vi "Draw Toolbar.vi"(8 "error in (no error)":errorcluster, 11 "Toolbar Control in":refnum<class "Toolbar Control.lvclass">) -> (0 "error out":errorcluster, 2 "Toolbar Image":picture, 3 "Toolbar Control out":refnum<class "Toolbar Control.lvclass">)   [LabVIEW 2011, in "Toolbar Control.lvclass"]
doc: "This VI will combine all the icons that are already drawn and return them on <B>Toolbar Image</B>.\n\n-------------\nDeveloped by Brian Hoover (hooovahh)"
uses:
  Toolbar Control.lvclass
  Toolbar Control.lvclass/Toolbar Control.ctl
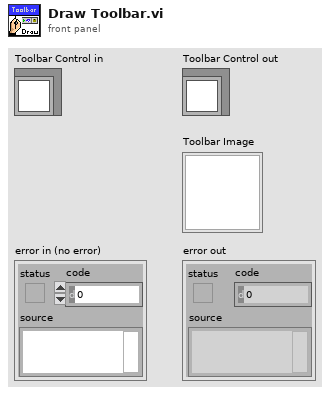
[diagram p1: front panel]
types:
  T1 = typedef "Toolbar Control.lvclass/Icon Data.ctl" = cluster{"Original Image Path":path, "Original Image Data":T2, "Scaled Icon":picture, "Button Name":string, "Button State":T3, "Icon Type":T4}
  T2 = typedef "imagedata.ctl" = cluster{"image type":i32, "image depth":i32, "image":u8[], "mask":u8[], "colors":u32[], "Rectangle":cluster{"left":i16, "top":i16, "right":i16, "bottom":i16}}
  T3 = typedef "Toolbar Control.lvclass/Button State.ctl" = enum8{"Enabled", "Disabled", "Disabled and Grayed Out"}
  T4 = typedef "Icon Type.ctl" = enum16{"Normal Icon", "Separator Icon", "More Options"}
  T5 = typedef "LVRectTypeDef.ctl" = cluster{"Left":i16, "Top":i16, "Right":i16, "Bottom":i16}
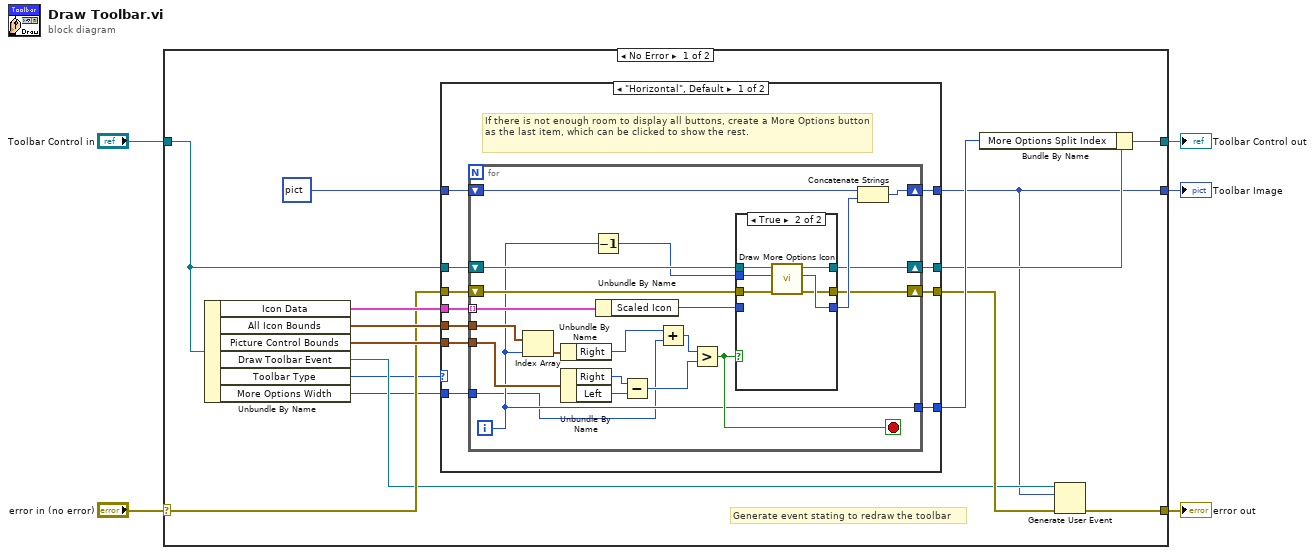
[diagram p0: block diagram]
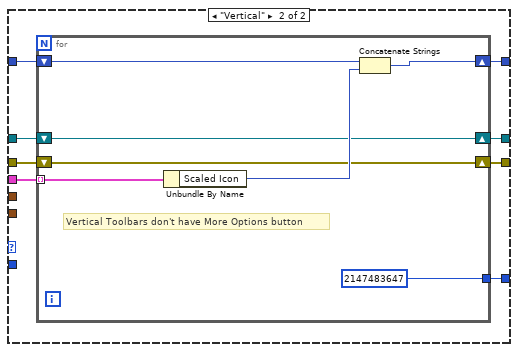
[diagram p3: hidden frame]
diagram:
  n1 = case shown="No Error" "error in (no error)" {
    selector: "error in (no error)" -> [w12 w78]
    tunnel: [w10 w78] -> w4
    tunnel: [w16 w77] -> w2
    tunnel: "Toolbar Control in" -> [w14 w77]
    tunnel: [w8 _] -> w1
    frame No Error {
      # "Generate event stating to redraw the toolbar"
      n2 = Unbundle By Name(w14) -> ("Icon Data"=w20:T1[], "All Icon Bounds"=w18:T5[], "Picture Control Bounds"=w17:T5, "Draw Toolbar Event"=w9:refnum<user-event>, "Toolbar Type"=w7:enum16{"Horizontal", "Vertical"}, "More Options Width"=w6:i32)
      n3 = case shown="\"Horizontal\", Default" w7 {
        tunnel: w20 -> [w31 w69]
        tunnel: picture data[5B] -> [w30 w68]
        tunnel: w18 -> [w29 _]
        tunnel: w17 -> [w28 _]
        tunnel: [w27 w62] -> w15
        tunnel: w14 -> [w26 w67]
        tunnel: [w25 w66] -> w13
        tunnel: w12 -> [w24 w65]
        tunnel: [w23 w64] -> w11
        tunnel: [w22 w63] -> w8
        tunnel: w6 -> [w21 _]
        frame "Horizontal", Default {
          # "If there is not enough room to display all buttons, create a More Options button as the last item, which can be clicked to show the rest."
          n4 = for {
            tunnel: w31 -> [w52] mode=indexing
            shift-right: [w51] -> w22
            shift-left: w30 -> [w50]
            tunnel: w29 -> [w49]
            tunnel: w28 -> [w47]
            tunnel: [w39] -> w27
            shift-right: [w42] -> w25
            shift-left: w26 -> [w43]
            shift-right: [w40] -> w23
            shift-left: w24 -> [w41]
            tunnel: w21 -> [w34]
            i -> [w39]
            stop <- w46 stop-if-true
            n5 = Index Array(array=w49, index=w39) -> (element=w48:T5)
            n6 = Unbundle By Name(w48) -> ("Right"=w33:i16)
            n7 = Unbundle By Name(w47) -> ("Right"=w37:i16, "Left"=w36:i16)
            n8 = Decrement(x=w39) -> (x-1=w38:i32)
            n9 = Unbundle By Name(w52) -> ("Scaled Icon"=w45:picture)
            n10 = Subtract(x=w37, y=w36) -> (x-y=w35:i16)
            n11 = Add(x=w33, y=w34) -> (x+y=w32:i32)
            n12 = Greater?(x=w32, y=w35) -> (0:w46:bool)
            n13 = case shown="True" w46 {
              tunnel: w45 -> [w55 _]
              tunnel: [w55 w59] -> w44
              tunnel: w43 -> [w54 w61]
              tunnel: [w54 w60] -> w42
              tunnel: w41 -> [w53 w58]
              tunnel: [w53 w57] -> w40
              tunnel: w38 -> [_ w56]
              frame False {
              }
              frame True {
                n14 = call "Draw More Options Icon.vi"("error in (no error)"=w58, "Index To Add"=w56, "Toolbar Control in"=w61) -> ("error out"=w57:errorcluster, "More Options Image"=w59:picture, "Toolbar Control out"=w60:refnum<class "Toolbar Control.lvclass">)  [unwired: 6 in]
              }
            }
            n15 = Concatenate Strings(w50, w44) -> (w51:picture)
          }
        }
        frame "Vertical" {
          n16 = for {
            tunnel: w69 -> [w76] mode=indexing
            shift-right: [w75] -> w63
            shift-left: w68 -> [w74]
            shift-right: [w72] -> w66
            shift-left: w67 -> [w72]
            shift-right: [w71] -> w64
            shift-left: w65 -> [w71]
            tunnel: [2147483647] -> w62
            # "Vertical Toolbars don't have More Options button"
            n17 = Unbundle By Name(w76) -> ("Scaled Icon"=w73:picture)
            n18 = Concatenate Strings(w74, w73) -> (w75:picture)
          }
        }
      }
      n19 = Bundle By Name(cluster=w13, "More Options Split Index"=w15) -> (w16:refnum<class "Toolbar Control.lvclass">)
      n20 = Generate User Event(user event=w9, event data cluster=w8, error in=w11) -> (error out=w10:errorcluster)  [unwired: 1 out]
    }
    frame Error {
    }
  }
  "error out" <- w4
  "Toolbar Control out" <- w2
  "Toolbar Image" <- w1
